vi "SENS_IF_FILT_SAMP_COUN.vi"(0 "VISA IN":refnum<visa-resource-name>, 1 "Count":i32, 5 "error in":errorcluster, 7 "Channel":i32) -> (14 "VISA Out":refnum<visa-resource-name>, 19 "error out":errorcluster)   [LabVIEW 2018, in "PNA-X.lvlib"]
doc: "SENSe<cnum>:IF:FILTer:SAMPle:COUNt <num> \n(Read-Write) Sets and returns the number of taps in the IF filter. The IF filter sample count setting is \nonly used when SENSe:IF:FILTer:SAMPle:COUNt:MODE is set to MANUAL. Critical Note: \nParameters \n<cnum> Existing channel number to manipulate. If unspecified, <cnum> is set to 1. \n<num> An integer value. (MIN and MAX return the minimum and maximum allowed values, \nrespectively.) \nExamples SENS:IF:FILT:SAMP:COUN 40 \nsense2:if:filter:sample:count maximum \nQuery Syntax SENS:IF:FILTer:SAMPle:COUNt? \nReturn Type Numeric \nDefault Instrument dependent."
uses:
  PNA-X.lvlib
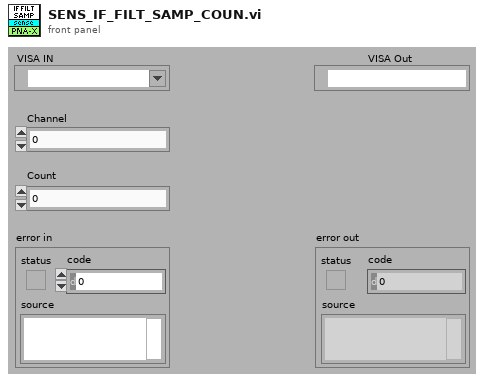
[diagram p1: front panel]
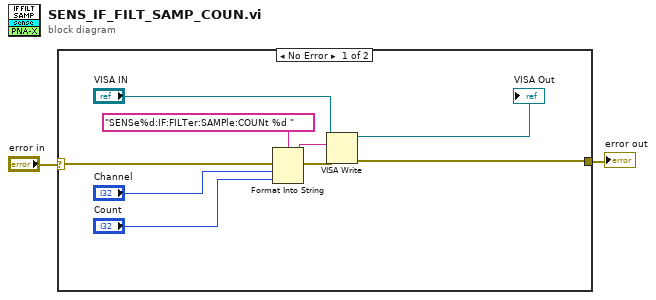
[diagram p0: block diagram]
diagram:
  n1 = case shown="No Error" "error in" {
    selector: "error in" -> [w11 w12]
    tunnel: [w3 w12] -> w1
    frame No Error {
      n2 = Format Into String(format string="SENSe%d:IF:FILTer:SAMPle:COUNt %d " ("Cmdline"), error in=w11, "Channel", "Count") -> (resulting string=w9:string, error out=w10:errorcluster)  [unwired: 1 in]
      n3 = VISA Write(VISA resource name="VISA IN", write buffer=w9, error in (no error)=w10) -> (VISA resource name out=→"VISA Out":refnum<visa-resource-name>, error out=w3:errorcluster)  [unwired: 1 out]
    }
    frame Error {
    }
  }
  "error out" <- w1
